vi "rp_error_structure.vi"(6 "Variant in":variant, 7 "Shift Pressed?":bool, 8 "error in (no error)":errorcluster, 10 "QD Combo Box Ref":refnum<vi>, 11 "QD Launch VI Ref":refnum<vi>) -> (0 "error out":errorcluster, 4 "Variant out":variant)   [LabVIEW 2019]
doc: "Wires the error terminals to the selected case structure and connects any unwired error cases. If the selector is already wired, this does nothing.\n\nCreated by: Ryan Pacini\n\nDefault Shortcut - [U]"
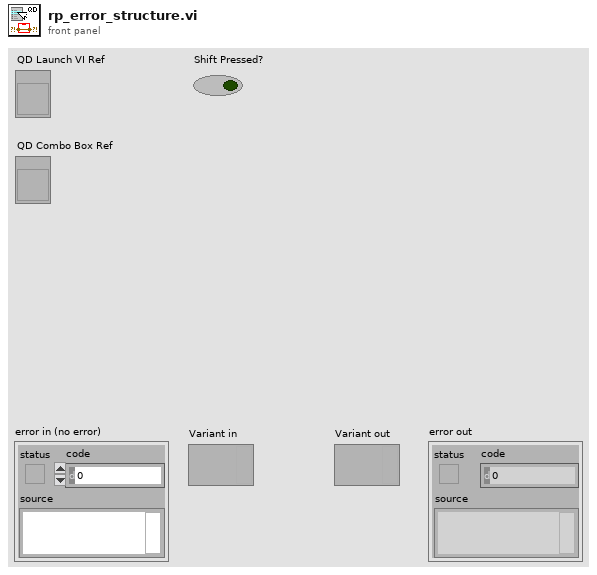
[diagram p1: front panel]
types:
  T1 = cluster{"in_tun":refnum<vi>, "in_term":refnum<vi>, "out_tun":refnum<vi>}
  T2 = typedef "LVPositionTypeDef.ctl" = cluster{"Left":i32, "Top":i32}
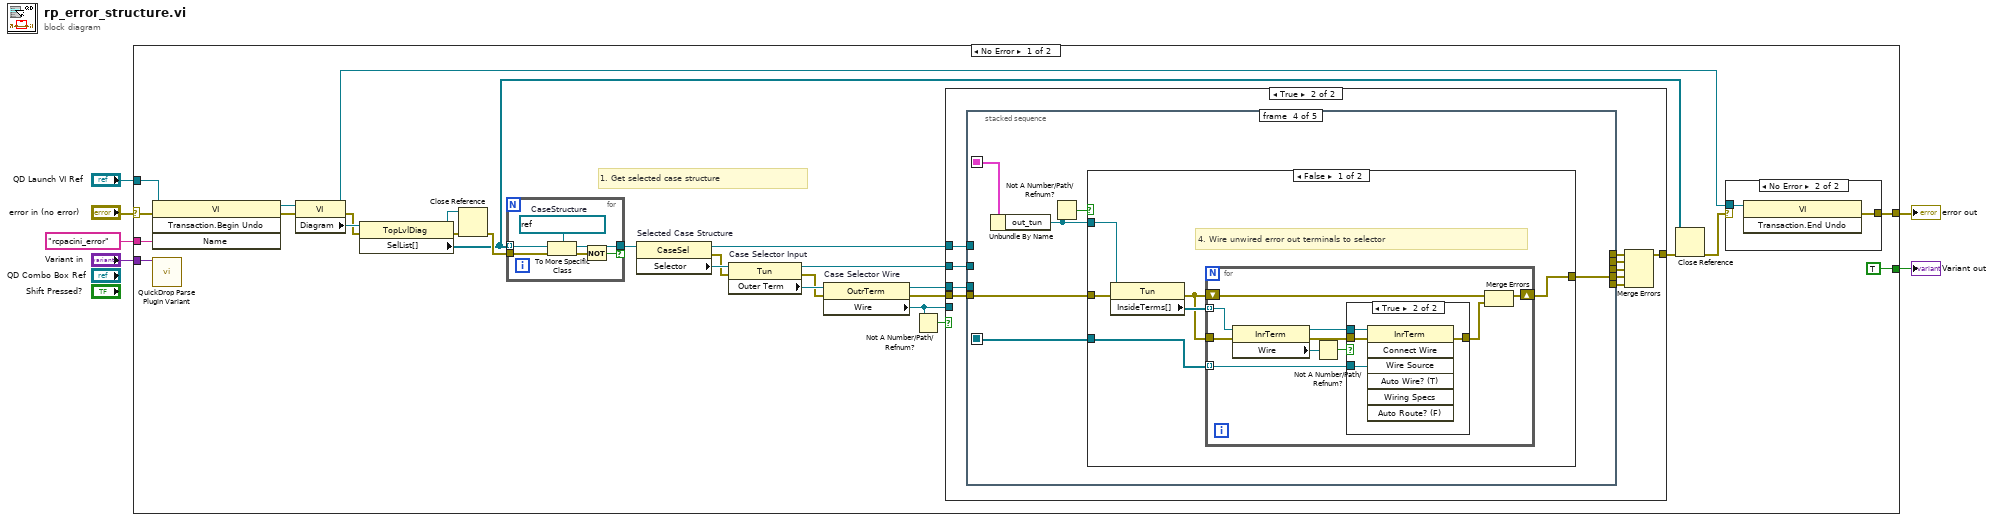
[diagram p0: block diagram]
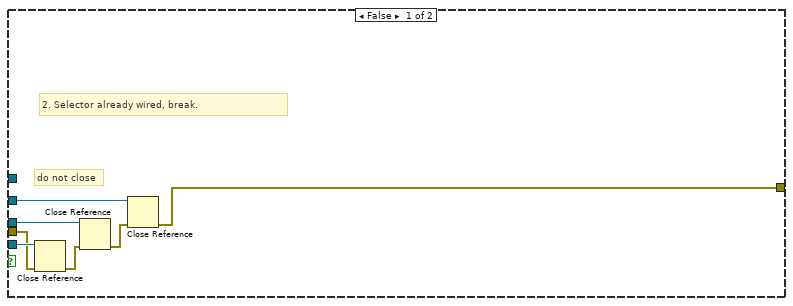
[diagram p2: hidden frame]
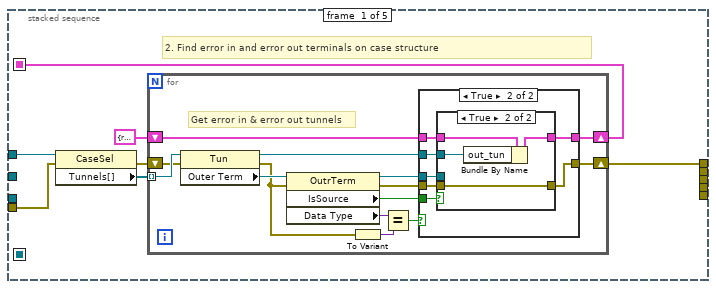
[diagram p3: hidden frame]
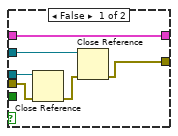
[diagram p4: hidden frame]
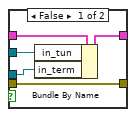
[diagram p5: hidden frame]
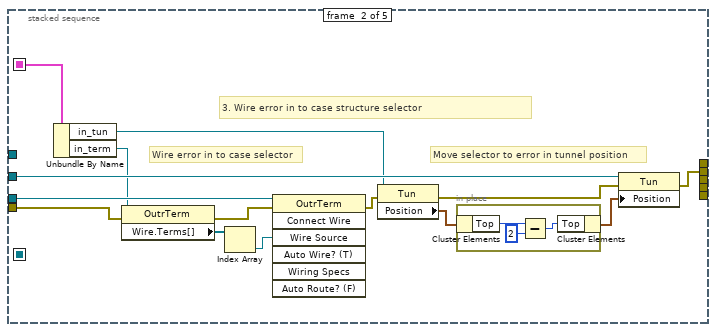
[diagram p6: hidden frame]
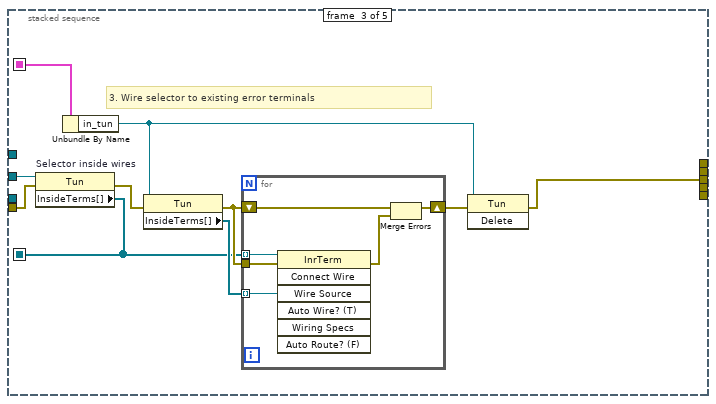
[diagram p7: hidden frame]
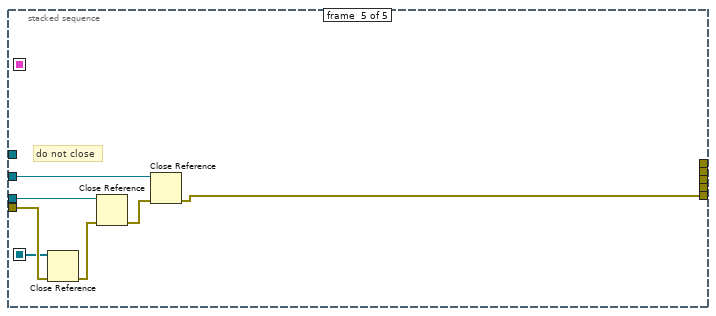
[diagram p10: hidden frame]
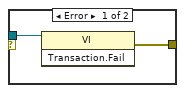
[diagram p11: hidden frame]
diagram:
  n1 = case shown="No Error" "error in (no error)" {
    selector: "error in (no error)" -> [w34 w173]
    tunnel: [w33 w173] -> w2
    tunnel: "QD Launch VI Ref" -> [w30 _]
    tunnel: "rcpacini_error" ("Undo Name") -> [w32 _]
    tunnel: [TRUE _] -> w3
    tunnel: "Variant in" -> [w29 _]
    frame No Error {
      # "1. Get selected case structure"
      n2 = invoke class="VI" method="Transaction.Begin Undo"(reference=w30, error in=w34, "Name"=w32) -> (reference out=w9:refnum<vi>, error out=w10:errorcluster)  [unwired: 1 in, 2 out]
      n3 = call <vilib>:"QuickDrop Parse Plugin Variant.vi"("QDKS Variant in"=w29) -> ()  [unwired: 12 in, 3 out]
      n4 = property class="VI"(reference=w9, error in=w10) -> (reference out=w8:refnum<vi>, error out=w24:errorcluster, "Diagram"=w28:refnum<vi>)
      n5 = property class="TopLvlDiag"(reference=w28, error in=w24) -> (reference out=w26:refnum<vi>, error out=w25:errorcluster, "SelList[]"=w23:refnum<vi>[])
      n6 = Close Reference(reference=w26, error in (no error)=w25) -> (error out=w27:errorcluster)
      n7 = for {
        tunnel: w23 -> [w167] mode=indexing
        tunnel: w27 -> [w168]
        tunnel: [w165] -> w22 if=w163
        w166 = refnum<vi> refnum  # CaseStructure
        n8 = To More Specific Class(target class=w166, reference=w167, error in=w168) -> (specific class reference=w165:refnum<vi>, error out=w164:errorcluster)
        n9 = Not(x=w164) -> (.not. x?=w163:bool)
      }
      n10 = property on="Selected Case Structure" class="CaseSel"(reference=w22) -> (reference out=w14:refnum<vi>, error out=w18:errorcluster, "Selector"=w21:refnum<vi>)  [unwired: 1 in]
      n11 = property on="Case Selector Input" class="Tun"(reference=w21, error in=w18) -> (reference out=w13:refnum<vi>, error out=w19:errorcluster, "Outer Term"=w20:refnum<vi>)
      n12 = property on="Case Selector Wire" class="OutrTerm"(reference=w20, error in=w19) -> (reference out=w12:refnum<vi>, error out=w15:errorcluster, "Wire"=w17:refnum<vi>)
      n13 = Not A Number/Path/Refnum?(number/path/refnum=w17) -> (NaN/Path/Refnum?=w16:bool)
      n14 = case shown="True" w16 {
        tunnel: w17 -> [w40 _]
        tunnel: w15 -> [w39 w50]
        tunnel: w14 -> [_ w51]
        tunnel: w13 -> [w41 w47]
        tunnel: w12 -> [w38 w46]
        tunnel: [w35 w48] -> w11
        frame False {
          # "2. Selector already wired, break."
          # "do not close"
          n15 = Close Reference(reference=w40, error in (no error)=w39) -> (error out=w37:errorcluster)
          n16 = Close Reference(reference=w38, error in (no error)=w37) -> (error out=w36:errorcluster)
          n17 = Close Reference(reference=w41, error in (no error)=w36) -> (error out=w35:errorcluster)
        }
        frame True {
          n18 = stacked-sequence {
            seq-local: [w53 _ _ _ _] -> [_ w108 w120 w132 _]
            seq-local: [_ _ w112 _ _] -> [_ _ _ w130 w156]
            tunnel: w51 -> [w55 _ _ _ _]
            tunnel: w50 -> [w54 w96 w115 w133 w162]
            tunnel: [w52 _ _ _ _] -> w49
            tunnel: w47 -> [_ w100 w113 _ w159]
            tunnel: w46 -> [_ w98 _ _ w161]
            tunnel: [_ w95 _ _ _] -> w45
            tunnel: [_ _ w116 _ _] -> w44
            tunnel: [_ _ _ w131 _] -> w43
            tunnel: [_ _ _ _ w157] -> w42
            frame #0 {
              # "2. Find error in and error out terminals on case structure"
              n19 = property class="CaseSel"(reference=w55, error in=w54) -> (error out=w57:errorcluster, "Tunnels[]"=w58:refnum<vi>[])  [unwired: 1 out]
              n20 = for {
                tunnel: w58 -> [w72] mode=indexing
                shift-right: [w63] -> w52
                shift-left: w57 -> [w71]
                shift-right: [w60] -> w53
                shift-left: T1 {"in_tun"=refnum, "in_term"=refnum, "out_tun"=refnum} ("ref") -> [w61]
                # "Get error in & error out tunnels"
                n21 = property class="Tun"(reference=w72, error in=w71) -> (reference out=w65:refnum<vi>, error out=w67:errorcluster, "Outer Term"=w70:refnum<vi>)
                n22 = property class="OutrTerm"(reference=w70, error in=w67) -> (reference out=w64:refnum<vi>, error out=w62:errorcluster, "IsSource"=w59:bool, "Data Type"=w69:variant)
                n23 = To Variant(anything=w67) -> (Variant=w68:variant)
                n24 = Equal?(x=w69, y=w68) -> (x = y?=w66:bool)
                n25 = case shown="True" w66 {
                  tunnel: w65 -> [w74 w84]
                  tunnel: w64 -> [w76 w83]
                  tunnel: [w75 w82] -> w63
                  tunnel: w62 -> [w78 w81]
                  tunnel: w59 -> [_ w85]
                  tunnel: w61 -> [w73 w80]
                  tunnel: [w73 w79] -> w60
                  frame False {
                    n26 = Close Reference(reference=w76, error in (no error)=w78) -> (error out=w77:errorcluster)
                    n27 = Close Reference(reference=w74, error in (no error)=w77) -> (error out=w75:errorcluster)
                  }
                  frame True {
                    n28 = case shown="True" w85 {
                      tunnel: w84 -> [w88 w93]
                      tunnel: w83 -> [w87 _]
                      tunnel: [w90 w94] -> w82
                      tunnel: w81 -> [w90 w94]
                      tunnel: w80 -> [w89 w92]
                      tunnel: [w86 w91] -> w79
                      frame False {
                        n29 = Bundle By Name(cluster=w89, "in_tun"=w88, "in_term"=w87) -> (w86:T1)
                      }
                      frame True {
                        n30 = Bundle By Name(cluster=w92, "out_tun"=w93) -> (w91:T1)
                      }
                    }
                  }
                }
              }
            }
            frame #1 {
              # "3. Wire error in to case structure selector"
              # "Move selector to error in tunnel position"
              # "Wire error in to case selector"
              n31 = Unbundle By Name(w108) -> ("in_tun"=w99:refnum<vi>, "in_term"=w97:refnum<vi>)
              n32 = property class="OutrTerm"(reference=w97, error in=w96) -> (error out=w103:errorcluster, "Wire.Terms[]"=w105:refnum<vi>[])  [unwired: 1 out]
              n33 = Index Array(array=w105) -> (element=w104:refnum<vi>)  [unwired: 1 in]
              n34 = invoke class="OutrTerm" method="Connect Wire"(reference=w98, error in=w103, "Wire Source"=w104) -> (error out=w107:errorcluster)  [unwired: 4 in, 6 out]
              n35 = property class="Tun"(reference=w99, error in=w107) -> (error out=w106:errorcluster, "Position"=w102:T2)  [unwired: 1 out]
              n36 = in-place {
                n37 = in-place-cluster #1(w102) -> ("Top"=w111:i32)
                n38 = Subtract(x=w111, y=2 ("x")) -> (x-y=w110:i32)
                n39 = in-place-cluster #1("Top"=w110) -> (w101:T2)
              }
              n40 = property class="Tun"(reference=w100, error in=w106, "Position"=w101) -> (error out=w95:errorcluster)  [unwired: 1 out]
            }
            frame #2 {
              # "3. Wire selector to existing error terminals"
              n41 = property on="Selector inside wires" class="Tun"(reference=w113, error in=w115) -> (error out=w114:errorcluster, "InsideTerms[]"=w112:refnum<vi>[])  [unwired: 1 out]
              n42 = Unbundle By Name(w120) -> ("in_tun"=w119:refnum<vi>)
              n43 = property class="Tun"(reference=w119, error in=w114) -> (error out=w118:errorcluster, "InsideTerms[]"=w121:refnum<vi>[])  [unwired: 1 out]
              n44 = for {
                tunnel: w118 -> [w127]
                tunnel: w112 -> [w125] mode=indexing
                tunnel: w121 -> [w124] mode=indexing
                shift-right: [w123] -> w117
                shift-left: w118 -> [w122]
                n45 = invoke class="InrTerm" method="Connect Wire"(reference=w125, error in=w127, "Wire Source"=w124) -> (error out=w126:errorcluster)  [unwired: 4 in, 6 out]
                n46 = Merge Errors(w122, w126) -> (w123:errorcluster)
              }
              n47 = invoke class="Tun" method="Delete"(reference=w119, error in=w117) -> (error out=w116:errorcluster)  [unwired: 1 in, 2 out]
            }
            frame #3 {
              n48 = Unbundle By Name(w132) -> ("out_tun"=w129:refnum<vi>)
              n49 = Not A Number/Path/Refnum?(number/path/refnum=w129) -> (NaN/Path/Refnum?=w128:bool)
              n50 = case shown="False" w128 {
                tunnel: w133 -> [w138 w155]
                tunnel: w129 -> [w137 _]
                tunnel: [w135 w155] -> w131
                tunnel: w130 -> [w134 _]
                frame False {
                  # "4. Wire unwired error out terminals to selector"
                  n51 = property class="Tun"(reference=w137, error in=w138) -> (error out=w136:errorcluster, "InsideTerms[]"=w139:refnum<vi>[])  [unwired: 1 out]
                  n52 = for {
                    tunnel: w139 -> [w148] mode=indexing
                    tunnel: w136 -> [w149]
                    tunnel: w134 -> [w143] mode=indexing
                    shift-right: [w141] -> w135
                    shift-left: w136 -> [w142]
                    n53 = property class="InrTerm"(reference=w148, error in=w149) -> (reference out=w144:refnum<vi>, error out=w145:errorcluster, "Wire"=w147:refnum<vi>)
                    n54 = Not A Number/Path/Refnum?(number/path/refnum=w147) -> (NaN/Path/Refnum?=w146:bool)
                    n55 = case shown="True" w146 {
                      tunnel: w145 -> [w150 w154]
                      tunnel: w144 -> [_ w153]
                      tunnel: w143 -> [_ w152]
                      tunnel: [w150 w151] -> w140
                      frame False {
                      }
                      frame True {
                        n56 = invoke class="InrTerm" method="Connect Wire"(reference=w153, error in=w154, "Wire Source"=w152) -> (error out=w151:errorcluster)  [unwired: 4 in, 6 out]
                      }
                    }
                    n57 = Merge Errors(w142, w140) -> (w141:errorcluster)
                  }
                }
                frame True {
                }
              }
            }
            frame #4 {
              # "do not close"
              n58 = Close Reference(reference=w156, error in (no error)=w162) -> (error out=w160:errorcluster)
              n59 = Close Reference(reference=w161, error in (no error)=w160) -> (error out=w158:errorcluster)
              n60 = Close Reference(reference=w159, error in (no error)=w158) -> (error out=w157:errorcluster)
            }
          }
          n61 = Merge Errors(w49, w45, w44, w43, w42) -> (w48:errorcluster)
        }
      }
      n62 = Close Reference(reference=w23, error in (no error)=w11) -> (error out=w7:errorcluster)
      n63 = case shown="No Error" w7 {
        tunnel: w8 -> [w169 w171]
        tunnel: [w170 w172] -> w33
        frame Error {
          n64 = invoke class="VI" method="Transaction.Fail"(reference=w169) -> (error out=w170:errorcluster)  [unwired: 2 in, 2 out]
        }
        frame No Error {
          n65 = invoke class="VI" method="Transaction.End Undo"(reference=w171) -> (error out=w172:errorcluster)  [unwired: 2 in, 2 out]
        }
      }
    }
    frame Error {
    }
  }
  "error out" <- w2
  "Variant out" <- w3
